vi "Read Logger.vi"(11 "Abstract PLC Controler in":refnum<class "Abstract PLC Controler.lvclass">) -> (2 "EventLogger.lvlibp:Logger.lvclass":refnum<class "Logger.lvclass">, 3 "Abstract PLC Controler out":refnum<class "Abstract PLC Controler.lvclass">)   [LabVIEW 2020, in "HslCommunication.lvlib" / "Abstract PLC Controler.lvclass"]
uses:
  Abstract PLC Controler.lvclass
  EventLogger.lvlibp/Logger.lvclass
  Abstract PLC Controler.lvclass/Abstract PLC Controler.ctl
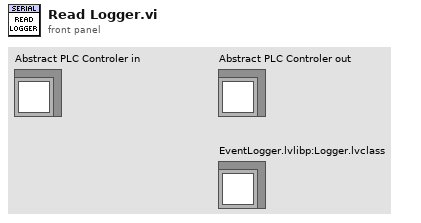
[diagram p1: front panel]
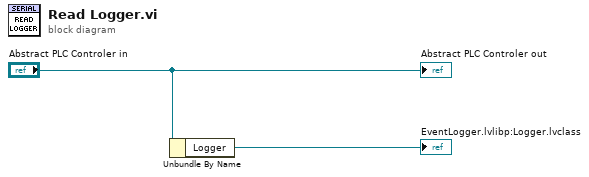
[diagram p0: block diagram]
diagram:
  n1 = Unbundle By Name("Abstract PLC Controler in") -> ("Logger"=→"EventLogger.lvlibp:Logger.lvclass":refnum<class "Logger.lvclass">)
  "Abstract PLC Controler out" <- "Abstract PLC Controler in"
